vi "File IsAlreadyOpen.vi"(8 "error in":errorcluster, 11 "file path (use dialog)":path) -> (0 "error out":errorcluster, 2 "already Open?":bool, 3 "file path (use dialog) (dup)":path)   [LabVIEW 2020, in "FileSync -- Base.lvlib" / "Protocol.lvclass"]
uses:
  Protocol.lvclass
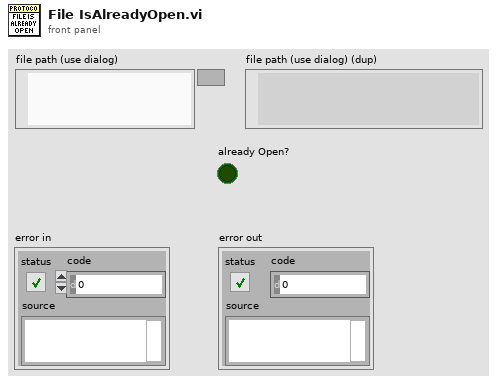
[diagram p1: front panel]
types:
  T1 = enum16{"open", "replace", "create", "open or create", "replace or create", "replace or create with confirmation"}
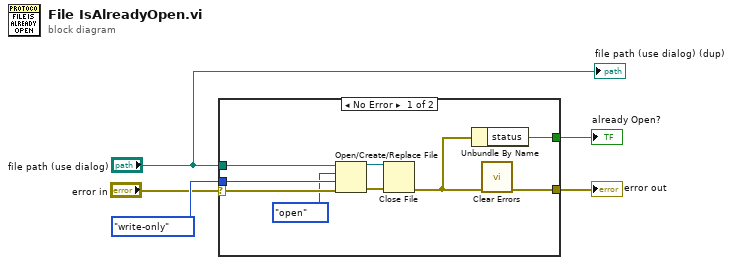
[diagram p0: block diagram]
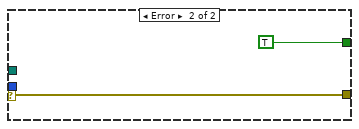
[diagram p2: hidden frame]
diagram:
  n1 = case shown="No Error" "error in" {
    selector: "error in" -> [w12 w16]
    tunnel: enum16{"read/write", "read-only", "write-only"}."write-only" ("access (0:read/write)") -> [w14 _]
    tunnel: "file path (use dialog)" -> [w13 _]
    tunnel: [w9 w16] -> w3
    tunnel: [w7 TRUE ("status")] -> w2
    frame No Error {
      n2 = Open/Create/Replace File(file path (use dialog)=w13, error in=w12, operation (0:open)=T1."open", access (0:read/write)=w14) -> (refnum out=w10:refnum<file>, error out=w11:errorcluster)  [unwired: 2 in, 1 out]
      n3 = Close File(refnum=w10, error in=w11) -> (error out=w8:errorcluster)  [unwired: 1 out]
      n4 = Unbundle By Name(w8) -> ("status"=w7:bool)
      n5 = call <vilib>:"Clear Errors.vi"("error in (no error)"=w8) -> ("error out"=w9:errorcluster)  [unwired: 5 in, 1 out]
    }
    frame Error {
    }
  }
  "error out" <- w3
  "already Open?" <- w2
  "file path (use dialog) (dup)" <- "file path (use dialog)"
